vi "Datalog file create v1.vi"(8 "error in (no error)":errorcluster) -> (0 "error out":errorcluster, 2 "File path out":path)   [LabVIEW 2017]
doc: "v1:\n- Added pressure 1 & 2 for logging"
uses:
  <vilib>/Utility/file.llb/Write Delimited Spreadsheet (string).vi
  GV/Specs.vi
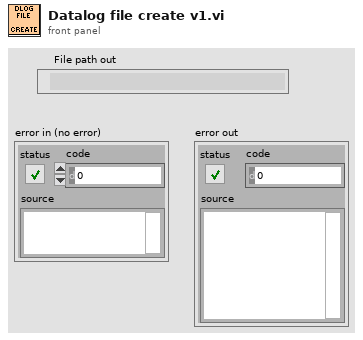
[diagram p1: front panel]
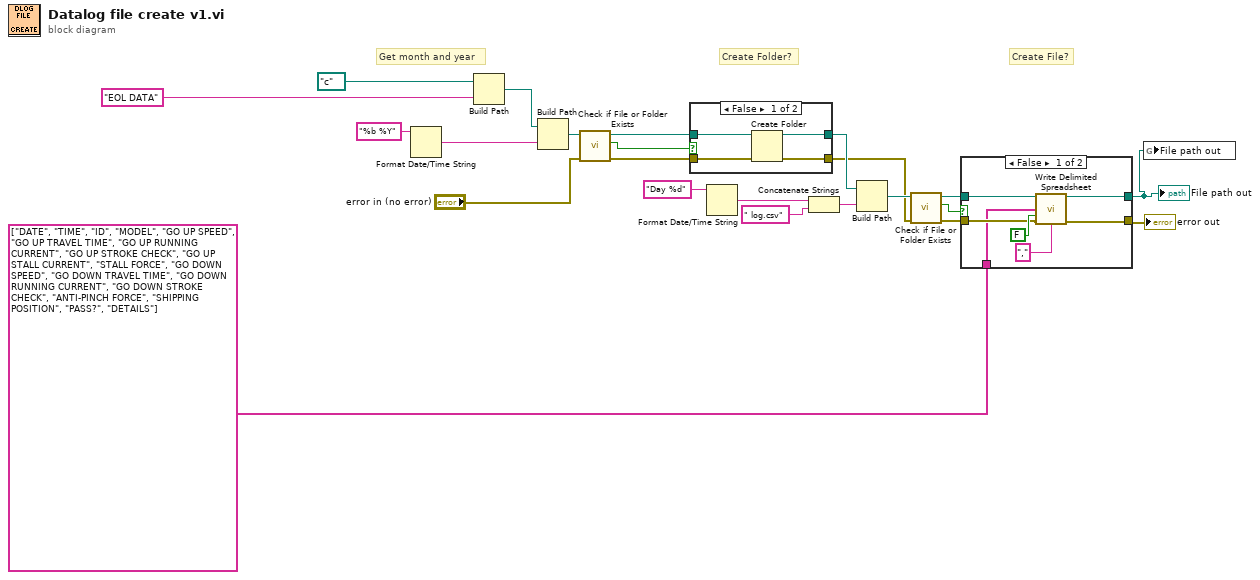
[diagram p0: block diagram]
diagram:
  # "Create File?"
  # "Create Folder?"
  # "Get month and year"
  n1 = Format Date/Time String(time format string (%c)="%b %Y") -> (date/time string=w16:string)  [unwired: 2 in]
  n2 = Build Path(base path=path "c:/", name or relative path="EOL DATA") -> (appended path=w7:path)
  n3 = Build Path(base path=w7, name or relative path=w16) -> (appended path=w15:path)
  n4 = call <vilib>:"Check if File or Folder Exists.vi"("error in (no error)"="error in (no error)", "path"=w15) -> ("error out"=w10:errorcluster, "file or folder exists?"=w18:bool, "dup path"=w19:path)  [unwired: 7 in]
  n5 = case shown="False" w18 {
    tunnel: w19 -> [w27 w29]
    tunnel: [w26 w29] -> w14
    tunnel: w10 -> [w25 w28]
    tunnel: [w24 w28] -> w9
    frame False {
      n6 = Create Folder(path (use dialog)=w27, error in=w25) -> (created path=w26:path, error out=w24:errorcluster)  [unwired: 1 in, 1 out]
    }
    frame True {
    }
  }
  n7 = Format Date/Time String(time format string (%c)="Day %d") -> (date/time string=w22:string)  [unwired: 2 in]
  n8 = Concatenate Strings(w22, " log.csv" ("name or relative path")) -> (w20:string)
  n9 = Build Path(base path=w14, name or relative path=w20) -> (appended path=w13:path)
  n10 = call <vilib>:"Check if File or Folder Exists.vi"("error in (no error)"=w9, "path"=w13) -> ("error out"=w8:errorcluster, "file or folder exists?"=w11:bool, "dup path"=w12:path)  [unwired: 7 in]
  n11 = case shown="False" w11 {
    tunnel: w12 -> [w36 w38]
    tunnel: [w30 w38] -> w4
    tunnel: [w33 w37] -> w1
    tunnel: w8 -> [w34 w37]
    tunnel: string[] ["DATE", "TIME", "ID", "MODEL", "GO UP SPEED", "GO UP TRAVEL TIME", "GO UP RUNNING CURRENT", "GO UP STROKE CHECK", "GO UP STALL CURRENT", "STALL FORCE", "GO DOWN SPEED", "GO DOWN TRAVEL TIME", "GO DOWN RUNNING CURRENT", "GO DOWN STROKE CHECK", "ANTI-PINCH FORCE", "SHIPPING POSITION", "PASS?", "DETAILS"] -> [w31 _]
    frame False {
      n12 = call-poly <vilib>:"Write Delimited Spreadsheet.vi"("file path (dialog if empty)"=w36, "1D data"=w31, "append to file? (new file:F)"=FALSE ("append to file? (F)"), "error in (no error)"=w34, "delimiter (\\t)"="," ("delimiter (\\t)")) -> ("new file path (Not A Path if cancelled)"=w30:path, "error out"=w33:errorcluster)  [unwired: 9 in]
    }
    frame True {
    }
  }
  "File path out" <- w4
  "error out" <- w1
  n13 = global write "Specs.vi" "File path out"(w4) -> ()
